vi "foo.vi"() -> ()   [LabVIEW 2014]
panel:
  in  "x":dbl=1.0 format="%#_13g"
  out "x+y":dbl
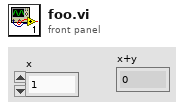
[diagram p1: front panel]
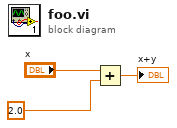
[diagram p0: block diagram]
diagram:
  n1 = Add(x="x", y=2.0) -> (x+y=→"x+y":dbl)
